vi "TestWrite0.vi"() -> ()   [LabVIEW 2021]
uses:
  <vilib>/MakerHub/LINX/Public/Peripherals/Digital/Digital Write 1 Chan.vi
  <vilib>/MakerHub/LINX/Public/Peripherals/Digital/Digital Write N Chans.vi
  <vilib>/MakerHub/LINX/Private/Local IO/LinxDigitalWrite.vi
  <vilib>/MakerHub/LINX/Public/Utilities/Check Channel.vi
  <vilib>/MakerHub/LINX/Public/Utilities/Open Serial.vi
  <vilib>/MakerHub/LINX/Private/Utilties/Generate Error.vi
  <vilib>/MakerHub/LINX/LMH-LINX.lvlib
panel:
  out "error out":errorcluster
  out "PIN Step":u8=11
  in  "Number of Steps":i32
  in  "DIR":bool
  out "PIN Direction":u8=12
  in  "Serial Port":refnum<visa-resource-name>="N/A"
  in  "M1":bool
  in  "M0":bool
  out "PIN M1":u8=9
  out "PIN M0":u8=8
  in  "Sleep":bool
  out "PIN Sleep":u8=10
  in  "error in (no error)":errorcluster
  # "Function & M0 & M1\n ----------------------\nFull  Step:       0         0\n1/2   Step:       1         0\n1/8   Step:       0         1\n1/16 Step:       1         1"
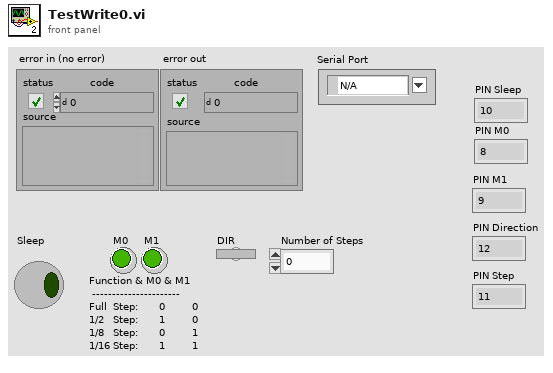
[diagram p1: front panel]
types:
  T1 = typedef "LMH-LINX.lvlib/LINX Ref.ctl" = cluster{"IO":T2, "Interface":T3, "LINX Device Config":T4}
  T2 = typedef "LMH-LINX.lvlib/Platform.ctl" = enum16{"Remote", "Local"}
  T3 = typedef "LMH-LINX.lvlib/Interface.ctl" = enum16{"Serial", "TCP"}
  T4 = typedef "LMH-LINX.lvlib/Device.lvlib/LINX Device Config.ctl" = cluster{"Interface":T3, "COM Port":refnum<visa-resource-name>, "TCP Configuration":T5, "Device Family":u8, "Device ID":u8, "Device Name":string, "TCP Ref":refnum<k5>, "Channels":T6}
  T5 = typedef "LMH-LINX.lvlib/Device.lvlib/TCP Config.ctl" = cluster{"IP Address":string, "Port":u16}
  T6 = typedef "LMH-LINX.lvlib/Channels.ctl" = cluster{"DI":u8[], "DO":u8[], "AI":u8[], "AO":u8[], "PWM":u8[], "QE":u8[], "UART":u8[], "I2C 2":u8[], "SPI":u8[], "CAN":u8[], "Servo":u8[], "AI Ref (V)":dbl, "AI Resolution (Bits)":u8, "AO Ref (V)":dbl, "AO Resolution (Bits)":u8}
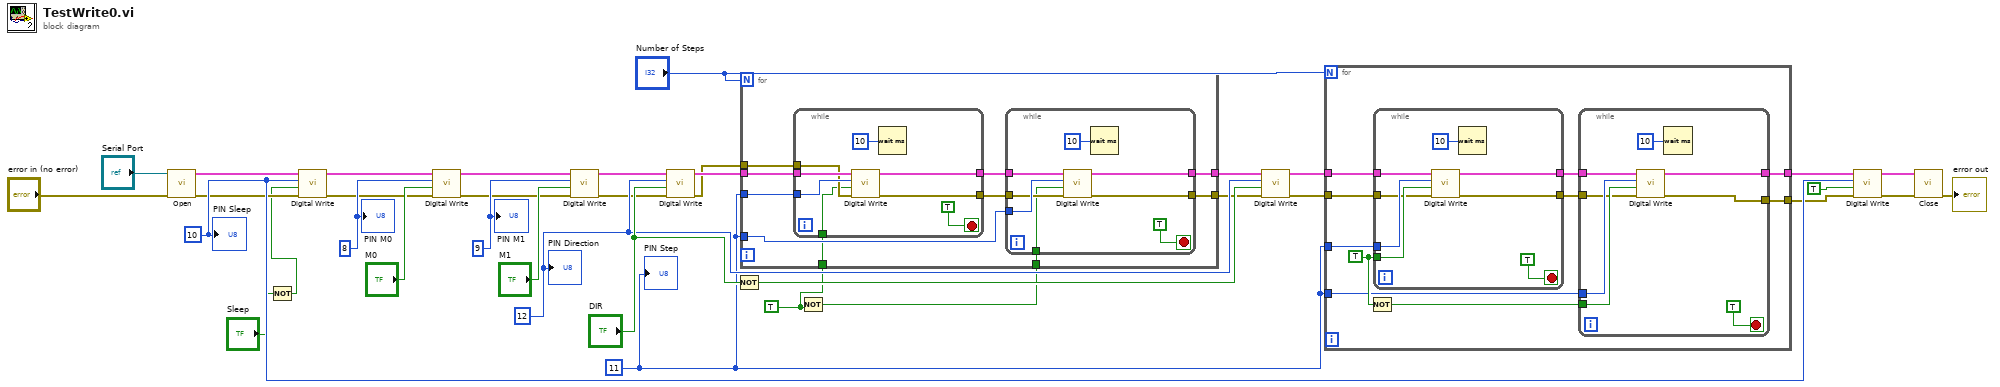
[diagram p0: block diagram]
diagram:
  w2 = TRUE ("Output Value")
  w21 = u8 11 ("DO Channel")
  w23 = u8 12 ("DO Channel")
  w31 = u8 9 ("DO Channel")
  w33 = u8 8 ("DO Channel")
  w18 = u8 10 ("DO Channel")
  n1 = call-poly <vilib>:"Open.vi"("Error In"="error in (no error)", "Serial Port"="Serial Port") -> ("Error Out"=w13:errorcluster, "LINX Resource"=w35:T1)  [unwired: 7 in, 1 out]
  n2 = Not(x="Sleep") -> (.not. x?=w3:bool)
  n3 = call-poly <vilib>:"Digital Write.vi"("Error In"=w13, "Output Value"=w3, "DO Channel"=w18, "LINX Resource"=w35) -> ("Error Out"=w12:errorcluster, "LINX Resource"=w34:T1)  [unwired: 6 in]
  n4 = call-poly <vilib>:"Digital Write.vi"("Error In"=w12, "Output Value"="M0", "DO Channel"=w33, "LINX Resource"=w34) -> ("Error Out"=w11:errorcluster, "LINX Resource"=w32:T1)  [unwired: 6 in]
  n5 = call-poly <vilib>:"Digital Write.vi"("Error In"=w11, "Output Value"="M1", "DO Channel"=w31, "LINX Resource"=w32) -> ("Error Out"=w10:errorcluster, "LINX Resource"=w27:T1)  [unwired: 6 in]
  n6 = call-poly <vilib>:"Digital Write.vi"("Error In"=w10, "Output Value"="DIR", "DO Channel"=w23, "LINX Resource"=w27) -> ("Error Out"=w9:errorcluster, "LINX Resource"=w25:T1)  [unwired: 6 in]
  n7 = Not(x="DIR") -> (.not. x?=w22:bool)
  n8 = Not(x=w2) -> (.not. x?=w1:bool)
  n9 = for {
    N: "Number of Steps" -> [_]
    tunnel: w25 -> [w46]
    tunnel: w21 -> [w45]
    tunnel: w21 -> [w44]
    tunnel: [w42] -> w24
    tunnel: w9 -> [w41]
    tunnel: [w39] -> w8
    tunnel: w2 -> [w38]
    tunnel: w1 -> [w37]
    n10 = while {
      tunnel: w46 -> [w62]
      tunnel: w45 -> [w61]
      tunnel: [w58] -> w43
      tunnel: w41 -> [w57]
      tunnel: [w56] -> w40
      tunnel: w38 -> [w55]
      stop <- TRUE stop-if-true
      n11 = call-poly <vilib>:"Digital Write.vi"("Error In"=w57, "Output Value"=w55, "DO Channel"=w61, "LINX Resource"=w62) -> ("Error Out"=w56:errorcluster, "LINX Resource"=w58:T1)  [unwired: 6 in]
      n12 = Wait (ms)(milliseconds to wait=u32 10) -> ()  [unwired: 1 out]
    }
    n13 = while {
      tunnel: w44 -> [w54]
      tunnel: w43 -> [w53]
      tunnel: [w50] -> w42
      tunnel: w40 -> [w49]
      tunnel: [w48] -> w39
      tunnel: w37 -> [w47]
      stop <- TRUE stop-if-true
      n14 = call-poly <vilib>:"Digital Write.vi"("Error In"=w49, "Output Value"=w47, "DO Channel"=w54, "LINX Resource"=w53) -> ("Error Out"=w48:errorcluster, "LINX Resource"=w50:T1)  [unwired: 6 in]
      n15 = Wait (ms)(milliseconds to wait=u32 10) -> ()  [unwired: 1 out]
    }
  }
  n16 = call-poly <vilib>:"Digital Write.vi"("Error In"=w8, "Output Value"=w22, "DO Channel"=w23, "LINX Resource"=w24) -> ("Error Out"=w7:errorcluster, "LINX Resource"=w20:T1)  [unwired: 6 in]
  n17 = for {
    N: "Number of Steps" -> [_]
    tunnel: w20 -> [w72]
    tunnel: w21 -> [w70]
    tunnel: w21 -> [w69]
    tunnel: [w66] -> w19
    tunnel: w7 -> [w65]
    tunnel: [w63] -> w6
    w71 = TRUE ("Output Value")
    n18 = Not(x=w71) -> (.not. x?=w68:bool)
    n19 = while {
      tunnel: w72 -> [w88]
      tunnel: w71 -> [w87]
      tunnel: w70 -> [w86]
      tunnel: [w83] -> w67
      tunnel: w65 -> [w82]
      tunnel: [w81] -> w64
      stop <- TRUE stop-if-true
      n20 = call-poly <vilib>:"Digital Write.vi"("Error In"=w82, "Output Value"=w87, "DO Channel"=w86, "LINX Resource"=w88) -> ("Error Out"=w81:errorcluster, "LINX Resource"=w83:T1)  [unwired: 6 in]
      n21 = Wait (ms)(milliseconds to wait=u32 10) -> ()  [unwired: 1 out]
    }
    n22 = while {
      tunnel: w69 -> [w80]
      tunnel: w68 -> [w79]
      tunnel: w67 -> [w78]
      tunnel: [w75] -> w66
      tunnel: w64 -> [w74]
      tunnel: [w73] -> w63
      stop <- TRUE stop-if-true
      n23 = call-poly <vilib>:"Digital Write.vi"("Error In"=w74, "Output Value"=w79, "DO Channel"=w80, "LINX Resource"=w78) -> ("Error Out"=w73:errorcluster, "LINX Resource"=w75:T1)  [unwired: 6 in]
      n24 = Wait (ms)(milliseconds to wait=u32 10) -> ()  [unwired: 1 out]
    }
  }
  n25 = call-poly <vilib>:"Digital Write.vi"("Error In"=w6, "Output Value"=TRUE, "DO Channel"=w18, "LINX Resource"=w19) -> ("Error Out"=w5:errorcluster, "LINX Resource"=w15:T1)  [unwired: 6 in]
  n26 = call <vilib>:"Close.vi"("Error In"=w5, "LINX Resource"=w15) -> ("Error Out"=→"error out":errorcluster)  [unwired: 9 in]
  "PIN Sleep" <- w18
  "PIN M0" <- w33
  "PIN M1" <- w31
  "PIN Direction" <- w23
  "PIN Step" <- w21
